vi "AttrMap-Preview.vi"(8 "error in (no error)":errorcluster, 11 "AttrMap in":T1) -> (0 "error out":errorcluster, 2 "data":variant, 3 "AttrMap out":T1)   [LabVIEW 2019]
uses:
  Typedef/Def-AttrMap.ctl
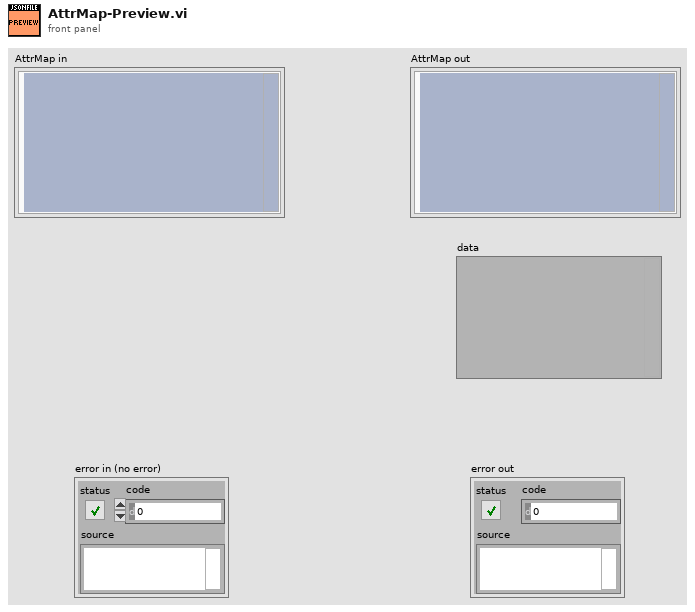
[diagram p1: front panel]
types:
  T1 = typedef "Def-AttrMap.ctl" = cluster{"Map":variant}
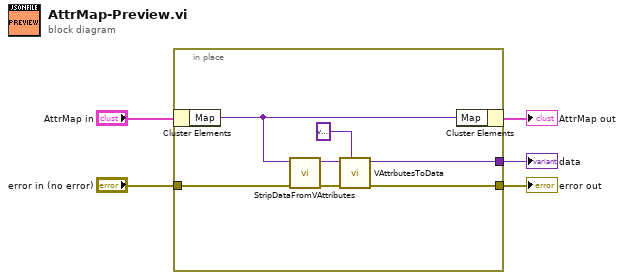
[diagram p0: block diagram]
diagram:
  n1 = in-place "In Place Element Structure" {
    in-place-border: [w11] -> w5
    in-place-border: "error in (no error)" -> [w7]
    in-place-border: [w10] -> w1
    n2 = in-place-cluster #1("AttrMap in") -> ("Map"=w12:variant)
    n3 = call "StripDataFromVAttributes.vi"("error in (no error)"=w7, "Map"=w12) -> ("error out"=w8:errorcluster, "duplicate variant"=w9:variant)  [unwired: 8 in]
    n4 = call "VAttrbutesToData.vi"("Prototype"=variant, "error in (no error)"=w8, "VAttributes"=w9) -> ("error out"=w11:errorcluster, "data"=w10:variant)  [unwired: 7 in]
    n5 = in-place-cluster #1("Map"=w12) -> (→"AttrMap out":T1)
  }
  "error out" <- w5
  "data" <- w1
